vi "Com_SECS Equipment _SECS Packet Read.vi"(8 "error in":errorcluster, 10 "Timeout(100)":i32=100, 11 "Buffer Data In":T5) -> (0 "error out":errorcluster, 1 "Timeout?":bool, 2 "SECS Packet":T1, 3 "Buffer Data Out":T5)   [LabVIEW 2016]
uses:
  Data Def/Com_SECS Equipment _Buffer Data.ctl
  Data Def/Com_SECS Equipment _Connection Setting.ctl
  Data Def/Com_SECS Equipment _Timeout Setting.ctl
  Data Def/Com_SECS Equipment _SECS Packet.ctl
  Data Def/Com_SECS Equipment _Message Type.ctl
  Data Def/Com_SECS Equipment _Protocol Type.ctl
  Data Def/Com_SECS Equipment _Stream Type.ctl
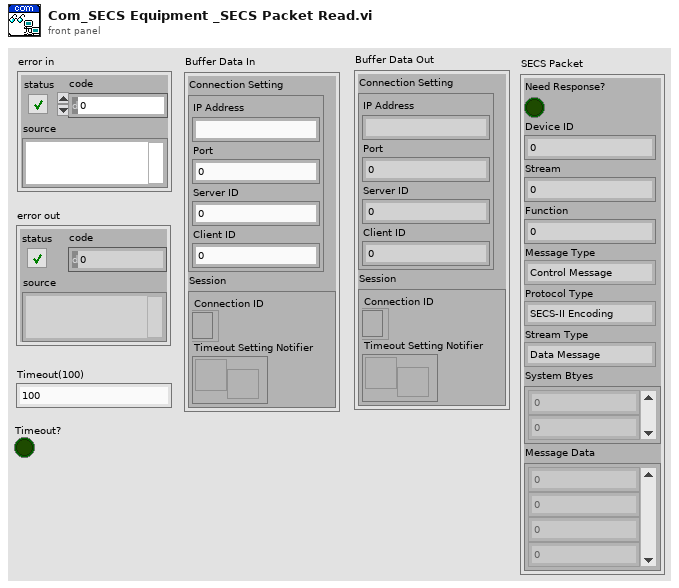
[diagram p1: front panel]
types:
  T1 = typedef "Com_SECS Equipment _SECS Packet.ctl" = cluster{"Need Response?":bool, "Device ID":u16, "Stream":u8, "Function":u8, "Message Type":T2, "Protocol Type":T3, "Stream Type":T4, "System Btyes":u8[], "Message Data":u8[]}
  T2 = typedef "Com_SECS Equipment _Message Type.ctl" = enum16{"Control Message", "Data Message"}
  T3 = typedef "Com_SECS Equipment _Protocol Type.ctl" = enum16{"SECS-II Encoding", "Reserved"}
  T4 = typedef "Com_SECS Equipment _Stream Type.ctl" = enum16{"Data Message", "Select.req", "Select.rsp", "Deselect.req", "Deselect.rsp", "Linktest.req", "Linktest.rsp", "Reject.req", "Separate.req", "Reserve"}
  T5 = typedef "Com_SECS Equipment _Buffer Data.ctl" = cluster{"Connection Setting":T6, "Session":cluster{"Connection ID":refnum<k5>, "Timeout Setting Notifier":refnum<notifier>}}
  T6 = typedef "Com_SECS Equipment _Connection Setting.ctl" = cluster{"IP Address":string, "Port":u16, "Server ID":u16, "Client ID":u16}
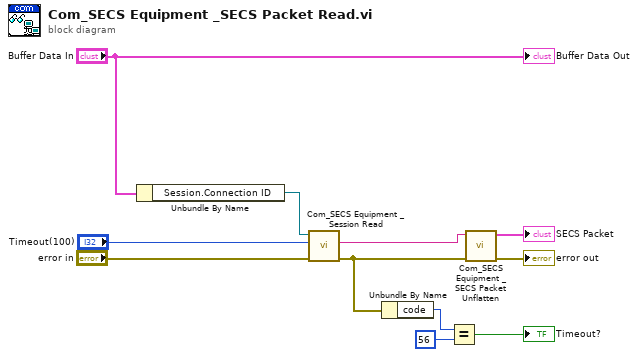
[diagram p0: block diagram]
diagram:
  n1 = Unbundle By Name("Buffer Data In") -> ("Session.Connection ID"=w11:refnum<k5>)
  n2 = call "Com_SECS Equipment _Session Read.vi"("error in"="error in", "Timeout(100)"="Timeout(100)", "Session In"=w11) -> ("error out"=w7:errorcluster, "Read Data"=w8:string)  [unwired: 6 in, 1 out]
  n3 = Unbundle By Name(w7) -> ("code"=w6:i32)
  n4 = Equal?(x=w6, y=56) -> (x = y?=→"Timeout?":bool)
  n5 = call "Com_SECS Equipment _SECS Packet Unflatten.vi"("error in"=w7, "Data"=w8) -> ("error out"=→"error out":errorcluster, "SECS Packet"=→"SECS Packet":T1)  [unwired: 8 in]
  "Buffer Data Out" <- "Buffer Data In"
